vi "Handle Error.vi"(8 "error in (no error)":errorcluster, 11 "ImageHandler in":refnum<class "ImageHandler.lvclass">) -> (0 "error out":errorcluster, 2 "stop actor?":bool=TRUE, 3 "ImageHandler out":refnum<class "ImageHandler.lvclass">)   [LabVIEW 2021, in "ImageHandler.lvlib" / "ImageHandler.lvclass"]
doc: "(<B>Filename</B>: Actor Framework.lvlib:Actor.lvclass:Handle Error.vi)\n\nDefines how the actor handles an error that occurred while processing a message.\n\nBy default, this method does nothing except stop the actor. This method also treats error code 43 (coming from <B>error in</B>) as a sign that the actor shut down normally. In this situation, the Handle Error method does not return the error on <B>error out</B>, meaning the actor's caller will not receive it. All other error codes will be returned on <B>error out</B>.\n\nA descendant class may override this method to change this behavior."
uses:
  ImageHandler.lvclass
  <vilib>/ActorFramework/Report Error Msg/Report Error Msg.lvclass
  <vilib>/ActorFramework/Actor/Actor.lvclass
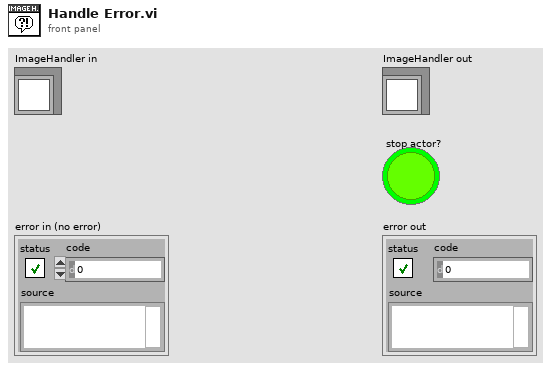
[diagram p1: front panel]
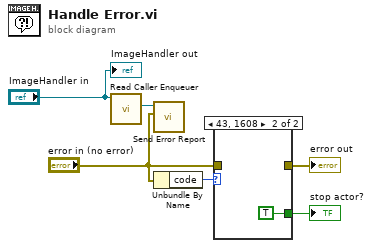
[diagram p0: block diagram]
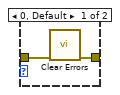
[diagram p2: hidden frame]
diagram:
  n1 = call <vilib>:"Read Caller Enqueuer.vi"("Actor"="ImageHandler in") -> ("Caller Enqueuer"=w6:refnum<class "Message Enqueuer.lvclass">)  [unwired: 10 in]
  n2 = call <vilib>:"Send Error Report.vi"("Error From Sender"="error in (no error)", "Message Enqueuer"=w6) -> ()  [unwired: 9 in, 1 out]
  n3 = Unbundle By Name("error in (no error)") -> ("code"=w4:i32)
  n4 = case shown="43, 1608" w4 {
    tunnel: [_ TRUE ("stop actor?")] -> w3
    tunnel: "error in (no error)" -> [w8 _]
    tunnel: [w7 _] -> w1
    frame 0, Default {
      n5 = call <vilib>:"Clear Errors.vi"("error in (no error)"=w8) -> ("error out"=w7:errorcluster)  [unwired: 5 in, 1 out]
    }
    frame 43, 1608 {
    }
  }
  "error out" <- w1
  "stop actor?" <- w3
  "ImageHandler out" <- "ImageHandler in"
